vi "Create TC Channels.vi"(8 "error in":errorcluster, 10 "Channel Data in":T3 {"Device Chan Total" max=32 step=1; "Thermocouple"."Temperature Units" items=["Celcius", "Fahrenheit", "Kelvin", "Rankine", "Volts"]; "Thermocouple"."Thermocouple Type" items=["J", "K", "T", "E", "N", "B", "R", "S", "Raw Voltage"]}, 11 "Device Configuration Data In":T1 {"Current Section Ref" format="%.0x"; "simTC Section Refs" format="%.0x"; "Voltage Section Ref" format="%.0x"; "Custom Device Ref" format="%.0x"}) -> (0 "error out":errorcluster, 2 "Channel Data Out":T3 {"Device Chan Total" max=32 step=1; "Thermocouple"."Temperature Units" items=["Celcius", "Fahrenheit", "Kelvin", "Rankine", "Volts"]; "Thermocouple"."Thermocouple Type" items=["J", "K", "T", "E", "N", "B", "R", "S", "Raw Voltage"]}, 3 "Device Configuration Data Out":T1 {"Current Section Ref" format="%.0x"; "simTC Section Refs" format="%.0x"; "Voltage Section Ref" format="%.0x"; "Custom Device Ref" format="%.0x"})   [LabVIEW 2011, in "Simulated Thermocouple Custom Device.lvlib"]
uses:
  Simulated Thermocouple Custom Device.lvlib
  New Channel Data.ctl
  TC Selector.ctl
  TC Unit Selector.ctl
  Device Config data.ctl
  <vilib>/NI Veristand/Custom Device API/Custom Device Item Ref.ctl
  TC Channel Config Data.ctl
  <vilib>/NI Veristand/Custom Device API/Custom Device Channel.ctl
  <vilib>/NI Veristand/Custom Device API/Custom Device Channel Type.ctl
  Calibration Config Data.ctl
  simTC Global GUIDs.vi
  <vilib>/NI Veristand/Custom Device Tools/Custom Device Utility Library/NI VeriStand - Search for Item by GUID.vi
  <vilib>/NI Veristand/Custom Device API/Set Item Property (Variant).vi
  <vilib>/NI Veristand/Custom Device API/Set Item Property (String).vi
  <vilib>/NI Veristand/Custom Device API/Get Item Property (Variant).vi
  <vilib>/NI Veristand/Custom Device API/Custom Device API.lvlib
  <vilib>/NI Veristand/Custom Device Tools/Custom Device Utility Library/Custom Device Utility Library.lvlib
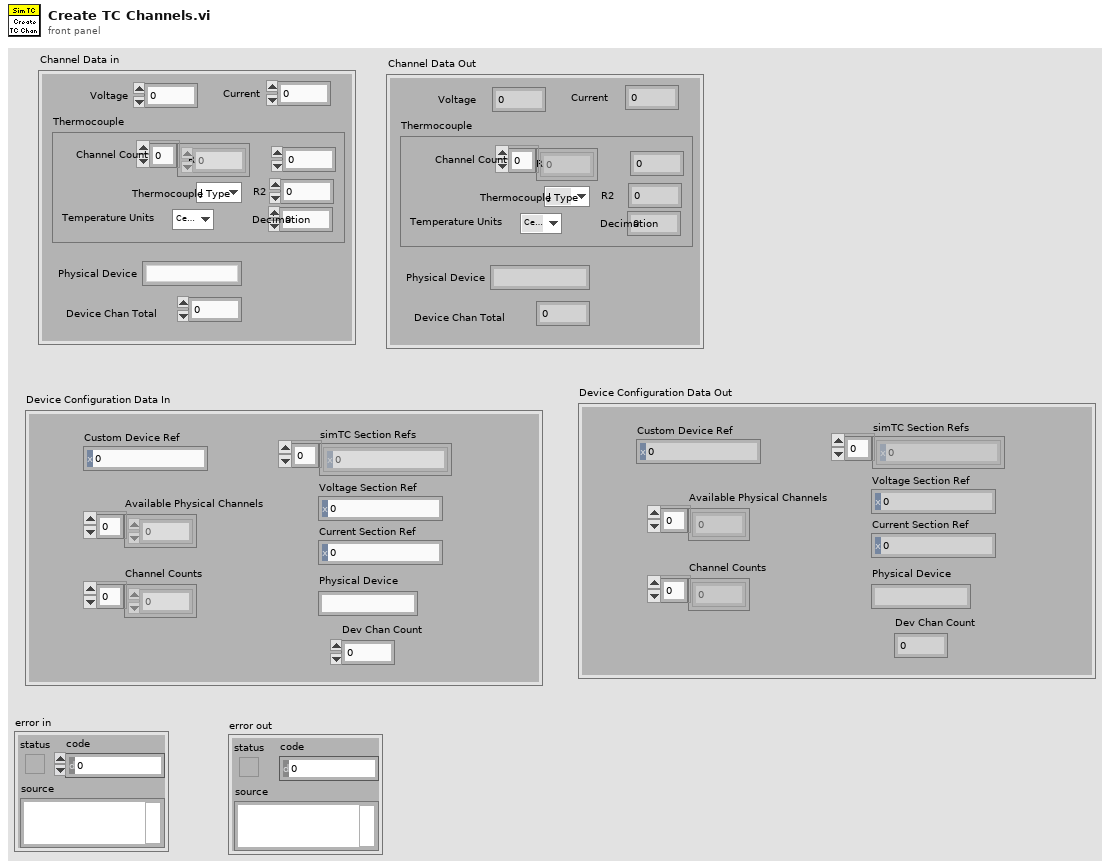
[diagram p1: front panel]
types:
  T1 = typedef "Simulated Thermocouple Custom Device.lvlib/Device Config data.ctl" = cluster{"Custom Device Ref":T2, "Voltage Section Ref":T2, "simTC Section Refs":T2[], "Current Section Ref":T2, "Physical Device":string, "Available Physical Channels":i32[], "Channel Counts":u32[], "Dev Chan Count":u32}
  T2 = typedef "Custom Device API.lvlib/Custom Device Item Ref.ctl" = u64
  T3 = typedef "Simulated Thermocouple Custom Device.lvlib/New Channel Data.ctl" = cluster{"Voltage":u32, "Current":u32, "Thermocouple":cluster{"R1":dbl, "R2":dbl, "Decimation":u32, "Thermocouple Type":T4, "Temperature Units":T5, "Channel Count":u32[]}, "Physical Device":string, "Device Chan Total":u32}
  T4 = typedef "Simulated Thermocouple Custom Device.lvlib/TC Selector.ctl" = u16
  T5 = typedef "Simulated Thermocouple Custom Device.lvlib/TC Unit Selector.ctl" = u16
  T6 = typedef "Simulated Thermocouple Custom Device.lvlib/TC Channel Config Data.ctl" = cluster{"Thermocouple Type":T4, "Temperature Units":T5}
  T7 = typedef "Custom Device API.lvlib/Custom Device Channel.ctl" = cluster{"Type":T8, "Units":string, "Default Value":dbl, "Faultable":bool, "Scalable":bool}
  T8 = typedef "Custom Device API.lvlib/Custom Device Channel Type.ctl" = enum16{"Input", "Output"}
  T9 = typedef "Simulated Thermocouple Custom Device.lvlib/Calibration Config Data.ctl" = cluster{"Local SimTC Chan":string, "Samples To Collect":dbl, "Cal Channel TC Type":T4, "Cal Step Settling Time":dbl}
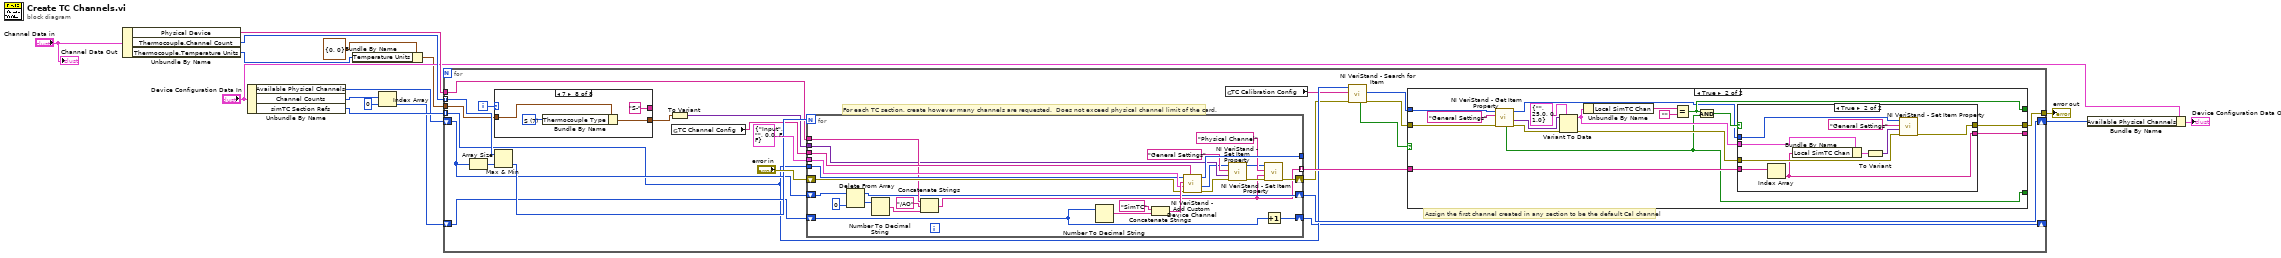
[diagram p0: block diagram]
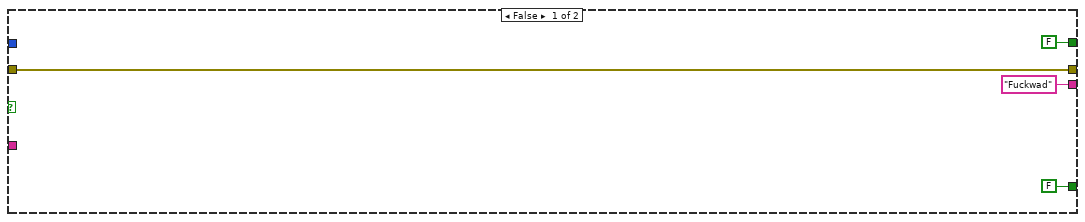
[diagram p2: hidden frame]
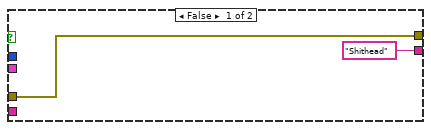
[diagram p3: hidden frame]
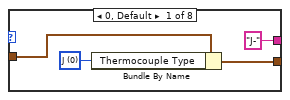
[diagram p4: hidden frame]
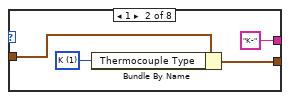
[diagram p5: hidden frame]
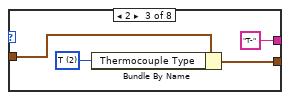
[diagram p6: hidden frame]
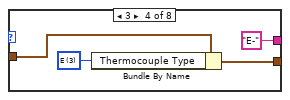
[diagram p7: hidden frame]
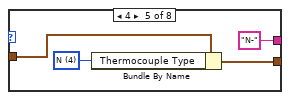
[diagram p8: hidden frame]
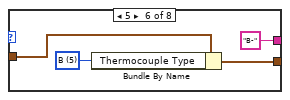
[diagram p9: hidden frame]
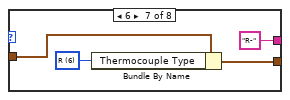
[diagram p10: hidden frame]
diagram:
  n1 = Unbundle By Name("Channel Data in") -> ("Physical Device"=w12:string, "Thermocouple.Channel Count"=w14:u32[], "Thermocouple.Temperature Units"=w6:T5)
  n2 = Unbundle By Name("Device Configuration Data In") -> ("Available Physical Channels"=w1:i32[], "Channel Counts"=w4:u32[], "simTC Section Refs"=w13:T2[])
  n3 = Bundle By Name(cluster=T6 {"Thermocouple Type"=0, "Temperature Units"=0} ("TC Channel Config"), "Temperature Units"=w6) -> (w5:T6)
  n4 = Index Array(array=w4, index=0) -> (element=w2:u32)
  n5 = for {
    tunnel: [w23] -> w15
    tunnel: w14 -> [w34] mode=indexing
    tunnel: w13 -> [w22] mode=indexing
    tunnel: w12 -> [w31]
    tunnel: w5 -> [w28]
    shift-right: [w29] -> w10
    shift-left: w1 -> [w32]
    shift-right: [w16] -> _
    shift-left: w2 -> [w25]
    i -> [w26]
    # "Assign the first channel created in any section to be the default Cal channel"
    # "For each TC section, create however many channels are requested.  Does not exceed physical channel limit of the card."
    n6 = Array Size(array=w32) -> (size(s)=w35:i32)
    n7 = case shown="7" w26 {
      tunnel: ["J-" "K-" "T-" "E-" "N-" "B-" "R-" "S-"] -> _
      tunnel: w28 -> [w71 w76 w80 w84 w87 w91 w96 w100]
      tunnel: [w73 w75 w79 w83 w88 w92 w95 w99] -> w27
      frame 0, Default {
        w72 = T4 0 items=["J", "K", "T", "E", "N", "B", "R", "S"] ("Cal Channel TC Type")
        n8 = Bundle By Name(cluster=w71, "Thermocouple Type"=w72) -> (w73:T6)
      }
      frame 1 {
        w77 = T4 1 items=["J", "K", "T", "E", "N", "B", "R", "S"] ("Cal Channel TC Type")
        n9 = Bundle By Name(cluster=w76, "Thermocouple Type"=w77) -> (w75:T6)
      }
      frame 2 {
        w81 = T4 2 items=["J", "K", "T", "E", "N", "B", "R", "S"] ("Cal Channel TC Type")
        n10 = Bundle By Name(cluster=w80, "Thermocouple Type"=w81) -> (w79:T6)
      }
      frame 3 {
        w85 = T4 3 items=["J", "K", "T", "E", "N", "B", "R", "S"] ("Cal Channel TC Type")
        n11 = Bundle By Name(cluster=w84, "Thermocouple Type"=w85) -> (w83:T6)
      }
      frame 4 {
        w89 = T4 4 items=["J", "K", "T", "E", "N", "B", "R", "S"] ("Cal Channel TC Type")
        n12 = Bundle By Name(cluster=w87, "Thermocouple Type"=w89) -> (w88:T6)
      }
      frame 5 {
        w93 = T4 5 items=["J", "K", "T", "E", "N", "B", "R", "S"] ("Cal Channel TC Type")
        n13 = Bundle By Name(cluster=w91, "Thermocouple Type"=w93) -> (w92:T6)
      }
      frame 6 {
        w97 = T4 6 items=["J", "K", "T", "E", "N", "B", "R", "S"] ("Cal Channel TC Type")
        n14 = Bundle By Name(cluster=w96, "Thermocouple Type"=w97) -> (w95:T6)
      }
      frame 7 {
        w101 = T4 7 items=["J", "K", "T", "E", "N", "B", "R", "S"] ("Cal Channel TC Type")
        n15 = Bundle By Name(cluster=w100, "Thermocouple Type"=w101) -> (w99:T6)
      }
    }
    n16 = Max & Min(x=w34, y=w35) -> (min(x,y)=w36:u32)  [unwired: 1 out]
    n17 = To Variant(anything=w27) -> (Variant=w30:variant)
    n18 = global read "simTC Global GUIDs.vi" "TC Channel Config"() -> (w33:string)
    n19 = for {
      N: w36 -> [_]
      tunnel: T7 {"Type"=enum."Input", "Units"="", "Default Value"=0.0, "Faultable"=FALSE, "Scalable"=FALSE} ("Channel") -> [w125]
      tunnel: w22 -> [w124]
      shift-right: [w108] -> w18
      shift-left: "error in" -> [w119]
      tunnel: [w123] -> _
      tunnel: w33 -> [w122]
      tunnel: w31 -> [w118]
      shift-right: [w116] -> w29
      shift-left: w32 -> [w107]
      tunnel: w30 -> [w114]
      tunnel: [w105] -> w24 mode=indexing
      shift-right: [w104] -> w16
      shift-left: w25 -> [w103]
      n20 = Delete From Array(array=w107, index=0) -> (deleted portion=w117:i32, array with subset deleted=w116:i32[])  [unwired: 1 in]
      n21 = Number To Decimal String(number=w117) -> (decimal integer string=w120:string)  [unwired: 1 in]
      n22 = Concatenate Strings(w118, "/AO", w120) -> (w105:string)
      n23 = Number To Decimal String(number=w103) -> (decimal integer string=w126:string)  [unwired: 1 in]
      n24 = Concatenate Strings("SimTC" ("Channel Name"), w126) -> (w128:string)
      n25 = call <vilib>:"NI VeriStand - Add Custom Device Channel.vi"("GUID (Default Channel)"=w122, "error in (no error)"=w119, "Channel"=w125, "Channel Name"=w128, "Parent Ref in"=w124) -> ("error out"=w115:errorcluster, "Channel Ref"=w112:T2, "Parent Ref out"=w123:T2)  [unwired: 3 in, 1 out]
      n26 = call-poly <vilib>:"NI VeriStand - Set Item Property.vi"("error in (no error)"=w115, "Value"=w114, "Property Name"="General Settings", "Item Ref in"=w112) -> ("error out"=w111:errorcluster, "Item Ref out"=w109:T2)  [unwired: 5 in, 1 out]
      n27 = call-poly <vilib>:"NI VeriStand - Set Item Property.vi"("error in (no error)"=w111, "Value"=w105, "Property Name"="Physical Channel", "Item Ref in"=w109) -> ("error out"=w108:errorcluster)  [unwired: 5 in, 2 out]
      n28 = Increment(x=w103) -> (x+1=w104:u32)
    }
    n29 = global read "simTC Global GUIDs.vi" "TC Calibration Config"() -> (w21:string)
    n30 = call-poly <vilib>:"NI VeriStand - Search for Item.vi"("error in"=w18, "Item GUID"=w21, "Section Ref in"=w22) -> ("error out"=w19:errorcluster, "Item Ref"=w20:T2, "Found"=w17:bool)  [unwired: 5 in, 1 out]
    n31 = case shown="True" w17 {
      tunnel: w24 -> [_ w54]
      tunnel: [w40 w52] -> w23
      tunnel: [FALSE w49] -> _
      tunnel: ["Fuckwad" w48] -> _
      tunnel: w20 -> [_ w47]
      tunnel: w19 -> [w40 w46]
      tunnel: [FALSE ("Found?") w44] -> _
      frame False {
      }
      frame True {
        n32 = call-poly <vilib>:"NI VeriStand - Get Item Property.vi"("error in (no error)"=w46, "Property Name"="General Settings", "Item Ref in"=w47) -> ("error out"=w58:errorcluster, "Value"=w56:variant, "Item Ref out"=w43:T2, "Found?"=w44:bool)  [unwired: 5 in]
        n33 = Variant To Data(error in=w58, type=T9 {"Local SimTC Chan"="", "Samples To Collect"=25.0, "Cal Channel TC Type"=0, "Cal Step Settling Time"=1.0} ("Cal Info"), Variant=w56) -> (data=w53:T9, error out=w45:errorcluster)
        n34 = Unbundle By Name(w53) -> ("Local SimTC Chan"=w50:string)
        n35 = Equal?(x=w50, y="") -> (x = y?=w49:bool)
        n36 = And(x=w49, y=w44) -> (x .and. y?=w51:bool)
        n37 = case shown="True" w51 {
          tunnel: w54 -> [_ w70]
          tunnel: w53 -> [_ w69]
          tunnel: w43 -> [_ w68]
          tunnel: w45 -> [w61 w65]
          tunnel: [w61 w64] -> w52
          tunnel: ["Shithead" w62] -> w48
          frame False {
          }
          frame True {
            n38 = Index Array(array=w70) -> (element=w62:string)  [unwired: 1 in]
            n39 = Bundle By Name(cluster=w69, "Local SimTC Chan"=w62) -> (w66:T9)
            n40 = To Variant(anything=w66) -> (Variant=w67:variant)
            n41 = call-poly <vilib>:"NI VeriStand - Set Item Property.vi"("error in (no error)"=w65, "Value"=w67, "Property Name"="General Settings", "Item Ref in"=w68) -> ("error out"=w64:errorcluster)  [unwired: 5 in, 2 out]
          }
        }
      }
    }
  }
  "error out" <- w15
  n42 = Bundle By Name(cluster="Device Configuration Data In", "Available Physical Channels"=w10) -> (→"Device Configuration Data Out":T1)
  "Channel Data Out" <- "Channel Data in"
